vi "String Integer.vi"() -> ()   [LabVIEW 2020, in "Tests.lvlib"]
uses:
  Tests.lvlib
  9900c4dc-c850-460c-946e-bfe9baca9f35.vi
  ee38d790-4272-4388-947c-0975de151472.vi
  f583e5a7-b460-46ae-97b7-bf538478c745.vi
panel:
  out "Array":cluster{"Key Type":string, "Value Type":i32}[](array[cluster])
  out "Value":i32
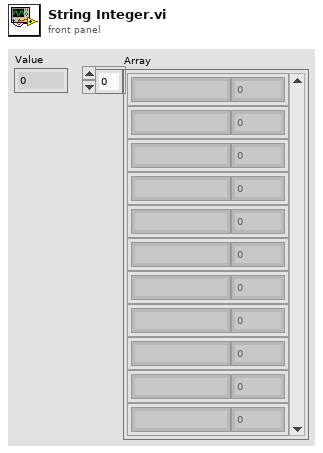
[diagram p1: front panel]
types:
  T1 = cluster{"Keys":string[], "Values":i32[], "Populated":bool[], "Lookup":map{string, i32}}
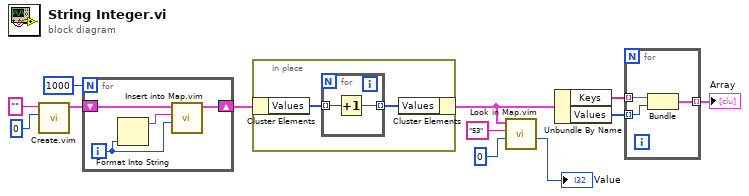
[diagram p0: block diagram]
diagram:
  n1 = call "Create.vim"("Value Type"=0, "Key Type"="") -> ("Iterable Map"=w12:T1)  [unwired: 6 in, 3 out]
  n2 = for {
    N: 1000 -> [_]
    shift-right: [w13] -> w8
    shift-left: w12 -> [w14]
    i -> [w15]
    n3 = Format Into String(w15) -> (resulting string=w16:string)  [unwired: 3 in, 1 out]
    n4 = call "Insert into Map.vim"("Value"=w15, "Key"=w16, "Iterable Map In"=w14) -> ("Iterable Map"=w13:T1)  [unwired: 7 in, 1 out]
  }
  n5 = in-place {
    n6 = in-place-cluster #1(w8) -> ("Values"=w18:i32[])
    n7 = for {
      tunnel: w18 -> [w20] mode=indexing
      tunnel: [w19] -> w17 mode=indexing
      n8 = Increment(x=w20) -> (x+1=w19:i32)
    }
    n9 = in-place-cluster #1("Values"=w17) -> (w5:T1)
  }
  n10 = call "Look in Map.vim"("Default Value"=0, "Key"="53", "Iterable Map In"=w5) -> ("Value"=→"Value":i32)  [unwired: 6 in, 2 out]
  n11 = Unbundle By Name(w5) -> ("Keys"=w4:string[], "Values"=w3:i32[])
  n12 = for {
    tunnel: w4 -> [w23] mode=indexing
    tunnel: w3 -> [w22] mode=indexing
    tunnel: [w21] -> w2 mode=indexing
    n13 = Bundle("Key Type"=w23, "Value Type"=w22) -> (w21:cluster{"Key Type":string, "Value Type":i32})  [unwired: 1 in]
  }
  "Array" <- w2
